vi "Config IQ Adjustments External.vi"(0 "VISA Resource Name":refnum<visa-resource-name>, 1 "Gain (0.0)":dbl format="%.2f", 2 "Attenuation Level (6.0)":dbl=6.0 format="%.2f", 5 "Common Offset (0.0)":dbl format="%.2f", 7 "I Differential Offset (0.0)":dbl format="%.2f", 9 "Q Differential Offset (0.0)":dbl format="%.2f", 11 "error in (no error)":errorcluster {"code" format="%.0x"}, 12 "I Offset (0.0)":dbl format="%.2f", 13 "Q Offset (0.0)":dbl format="%.2f") -> (4 "VISA Resource Name Out":refnum<visa-resource-name>, 15 "error out":errorcluster {"code" format="%.0x"})   [LabVIEW 2012, in "Agilent ESG Series.lvlib"]
doc: "This VI is used to set the External I/Q adjustments.\n\nNotes:\n(1) This VI is forAgilent E4438C instrument only."
uses:
  <instrlib>/Agilent ESG Series/Agilent ESG Series.lvlib
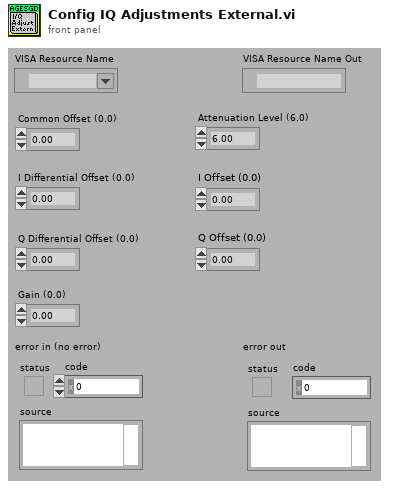
[diagram p1: front panel]
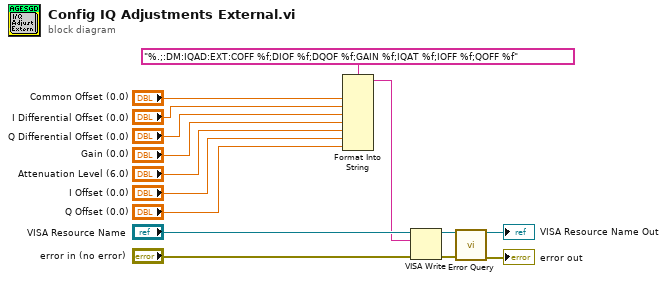
[diagram p0: block diagram]
diagram:
  n1 = Format Into String(format string="%.;:DM:IQAD:EXT:COFF %f;DIOF %f;DQOF %f;GAIN %f;IQAT %f;IOFF %f;QOFF %f", "Common Offset (0.0)", "I Differential Offset (0.0)", "Q Differential Offset (0.0)", "Gain (0.0)", "Attenuation Level (6.0)", "I Offset (0.0)", "Q Offset (0.0)") -> (resulting string=w12:string)  [unwired: 2 in, 1 out]
  n2 = VISA Write(VISA resource name="VISA Resource Name", write buffer=w12, error in (no error)="error in (no error)") -> (VISA resource name out=w4:refnum<visa-resource-name>, error out=w3:errorcluster)  [unwired: 1 out]
  n3 = call <instrlib>:"Error Query.vi"("VISA Resource Name"=w4, "error in (no error)"=w3) -> ("VISA Resource Name Out"=→"VISA Resource Name Out":refnum<visa-resource-name>, "error out"=→"error out":errorcluster)  [unwired: 10 in, 2 out]
